vi "Buttons View.vi"() -> ()   [LabVIEW 2015]
panel:
  in  "Button Light Minimize":bool
  in  "Button Light Close":bool
  in  "Button Light Maximize":bool
  in  "Button Add":bool
  in  "Button Calendar":bool
  in  "Button Line Chart":bool
  in  "Button Tool":bool
  in  "Button Calibration":bool
  in  "Button Mail":bool
  in  "Button QR Code":bool
  in  "Button USB":bool
  in  "Button Create Folder":bool
  in  "Button Play-Stop":bool
  in  "Button File":bool
  in  "Button Error":bool
  in  "Button Print":bool
  in  "Button Arrow Down":bool
  in  "Button Arrow Up":bool
  in  "Button Arrow Right":bool
  in  "Button Arrow Left":bool
  in  "Button Sync":bool
  in  "Button More Vertical":bool
  in  "Button More Horizontal":bool
  in  "Button Upload":bool
  in  "Button Edit":bool
  in  "Button Zoom Out":bool
  in  "Button Zoom In":bool
  in  "Button Report":bool
  in  "Button Delete":bool
  in  "Button Download":bool
  in  "Button Help Outline":bool
  in  "Button Settings":bool
  in  "Button Info":bool
  in  "Button Help":bool
  in  "Button GPS":bool
  in  "Button Folder 2":bool
  in  "Button Dark Play-Stop":bool
  in  "Button Dark USB":bool
  in  "Button Dark QR Code":bool
  in  "Button Dark Print":bool
  in  "Button Dark Mail":bool
  in  "Button Dark File":bool
  in  "Button Dark Error":bool
  in  "Button Dark Create Folder":bool
  in  "Button Dark Zoom Out":bool
  in  "Button Dark Zoom In":bool
  in  "Button Dark Upload":bool
  in  "Button Dark Sync":bool
  in  "Button Dark Report":bool
  in  "Button Dark More Vertical":bool
  in  "Button Dark More Horizontal":bool
  in  "Button Dark Edit":bool
  in  "Button Dark Tune":bool
  in  "Button Dark Tool":bool
  in  "Button Dark Minimize":bool
  in  "Button Dark Maximize":bool
  in  "Button Dark Line Chart":bool
  in  "Button Dark Close":bool
  in  "Button Dark Calendar":bool
  in  "Button Dark Add":bool
  in  "Button Dark Settings":bool
  in  "Button Dark Info":bool
  in  "Button Dark Help":bool
  in  "Button Dark Help Outline":bool
  in  "Button Dark GPS":bool
  in  "Button Dark Folder":bool
  in  "Button Dark Download":bool
  in  "Button Dark Delete":bool
  in  "Button Dark Arrow Up":bool
  in  "Button Dark Arrow Right":bool
  in  "Button Dark Arrow Left":bool
  in  "Button Dark Arrow Down":bool
  # "LabVIEW Material Light Icon Pack"
  # "Designed By Erencan TAYANÇ"
  # "LabVIEW Material Dark Icon Pack"
  # "Designed By Erencan TAYANÇ"
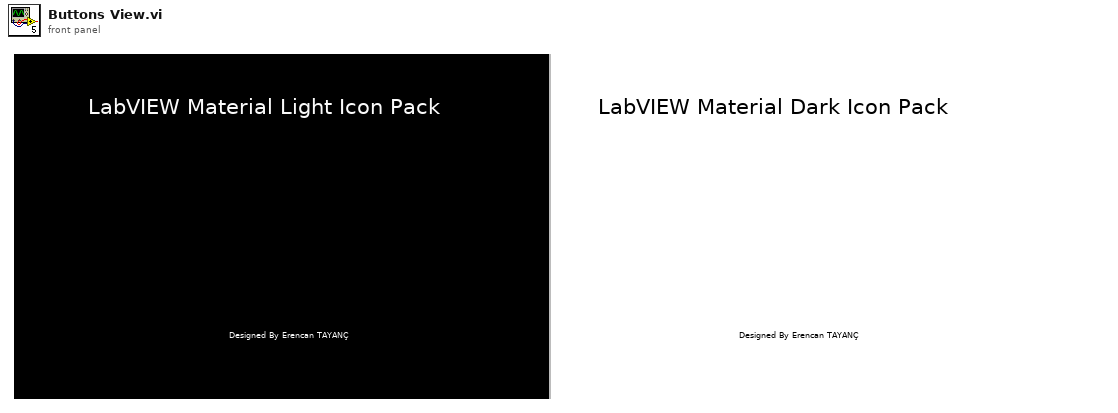
[diagram p1: front panel]
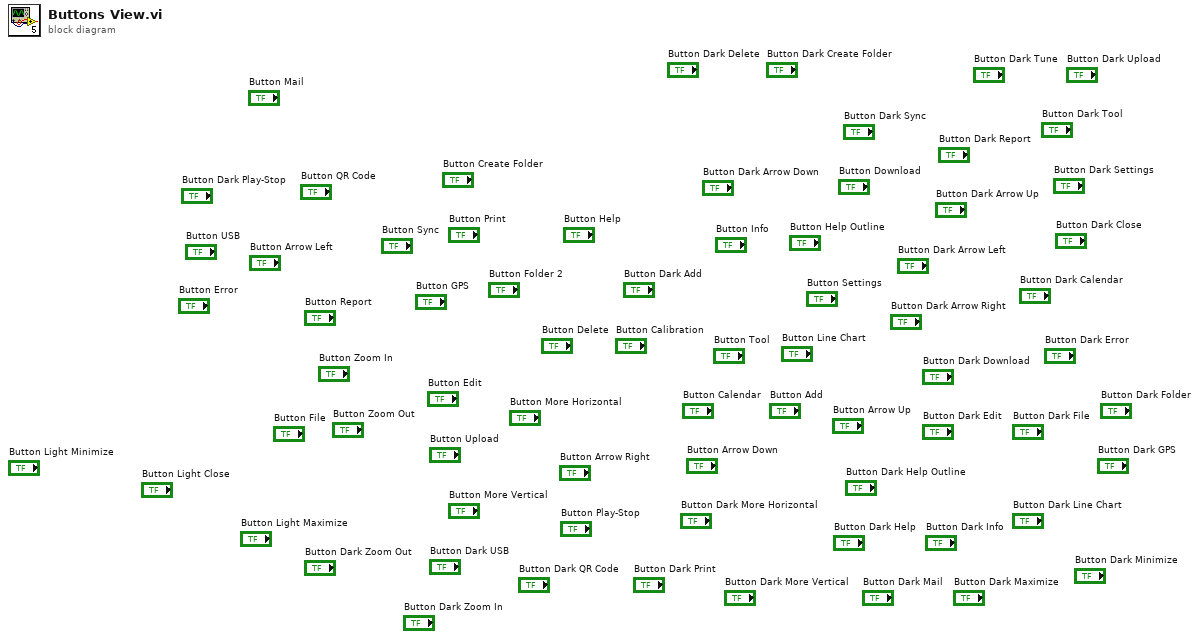
[diagram p0: block diagram]
diagram:
